vi "derivative_data view.vi"(8 "Y-column names":string[](array[string])=["col0"], 10 "column extension":string[](array[string])=["SCM1_2020Aug_AC.008.txt"], 11 "Graph array":cluster{"output":dbl[], "output":dbl[]}[](array[cluster])=[{"output"=array[450 elements], "output"=array[450 elements]}]) -> ()   [LabVIEW 2021]
uses:
  <vilib>/Analysis/1siggen.llb/Ramp Pattern by Samples.vi
  <vilib>/Analysis/NI_AALBase.lvlib
  <vilib>/gmath/NI_Gmath.lvlib
  <vilib>/Analysis/NI_AALPro.lvlib
panel:
  in  "iteration Number":i32=2
  in  "smooth factor":i32=121
  in  "method":u16(ring)=2 items=["2nd Order Central", "4th Order Central", "Forward", "Backward"]
  out "error code":i32
  out "bkg and subtracted data":cluster{"xi used":dbl[], "Integral X":dbl[]}[](graph)
  in  "remove bkg":bool=TRUE
  in  "Bbkg final":dbl=5.0 format="%.2f"
  in  "Bbkg initial":dbl=4.0 format="%.2f"
  in  "poly. order":i32=2
  in  "bkg removal method":enum16{"polynomial", "Cheby poly"}(ring)
  in  "export":T1(ring)=enum."write to clipboard"
  out "raw data":T2(graph)
  in  "interpol. method":i32(ring)=2 items=["nearest", "linear", "spline", "cubic Hermite", "Lagrange"]
  in  "stop":bool
  in  "use variables":bool
  in  "Interpolation #":i32=5000
  in  "export data":bool
  in  "smoothing factor":i32=3
  in  "final":dbl=5.0 format="%.2f"
  in  "init":dbl format="%.2f"
  out "dy/dx":cluster{"xi used":dbl[], "smoothed":dbl[]}[](graph)
  in  "variable":string="4.2\n3.5\n3"
  # "(0) Data are clipped defined by the 'init' and 'final'.\n(1) Boxcar averaging (use 'smoothing factor' for adjustment)\n(3) Background removal if necessary. Background removal is done by polynomial (normal or Chebychev).\n            i) fitting is done for the range given by 'Bbkg init' and 'Bbkg final'.\n            ii) the background curve is extended to the whole data range."
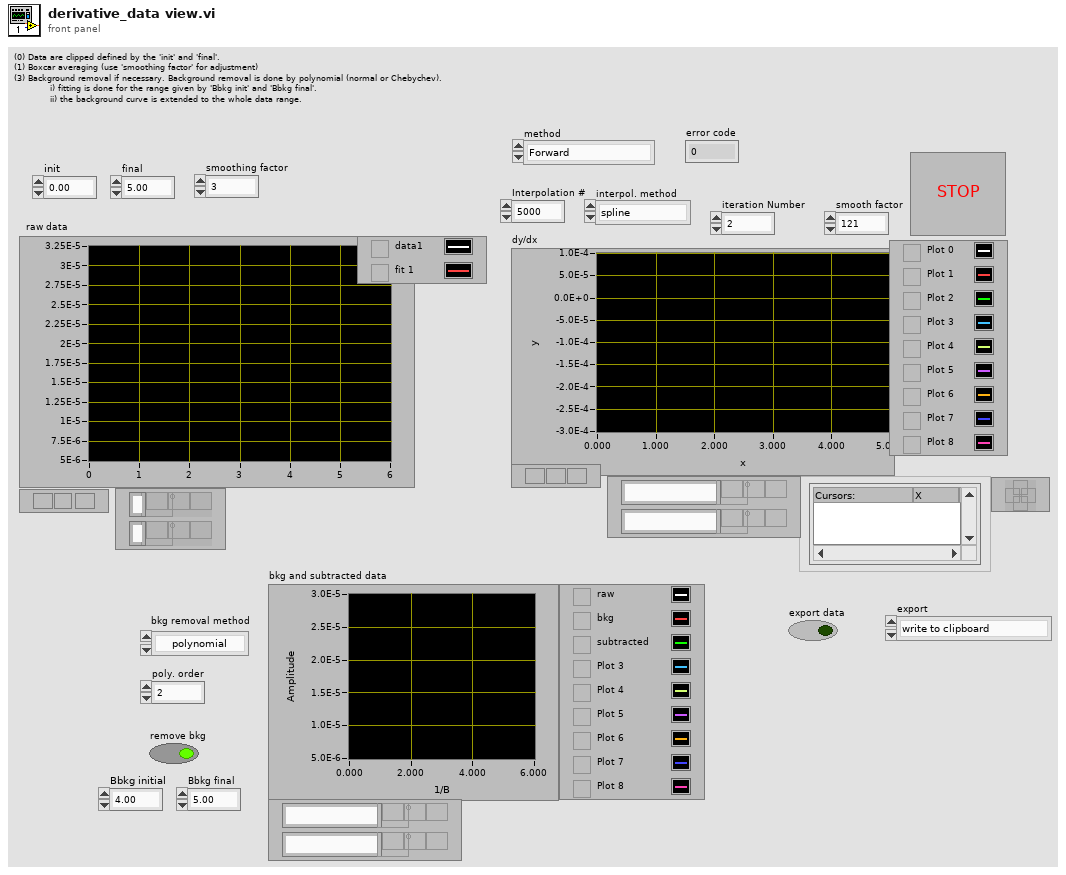
[diagram p1: front panel]
types:
  T1 = enum16{"Save as Ascill file", "write to clipboard", "write to Igor ITX file"}
  T2 = cluster{"Ramp Pattern":dbl[], "Power Spectrum":dbl[]}[]
  T3 = enum16{"Save as Ascill file", "write to clipboard", "do not export"}
  T4 = cluster{"all rows":dbl[], "extended data":dbl[]}[]
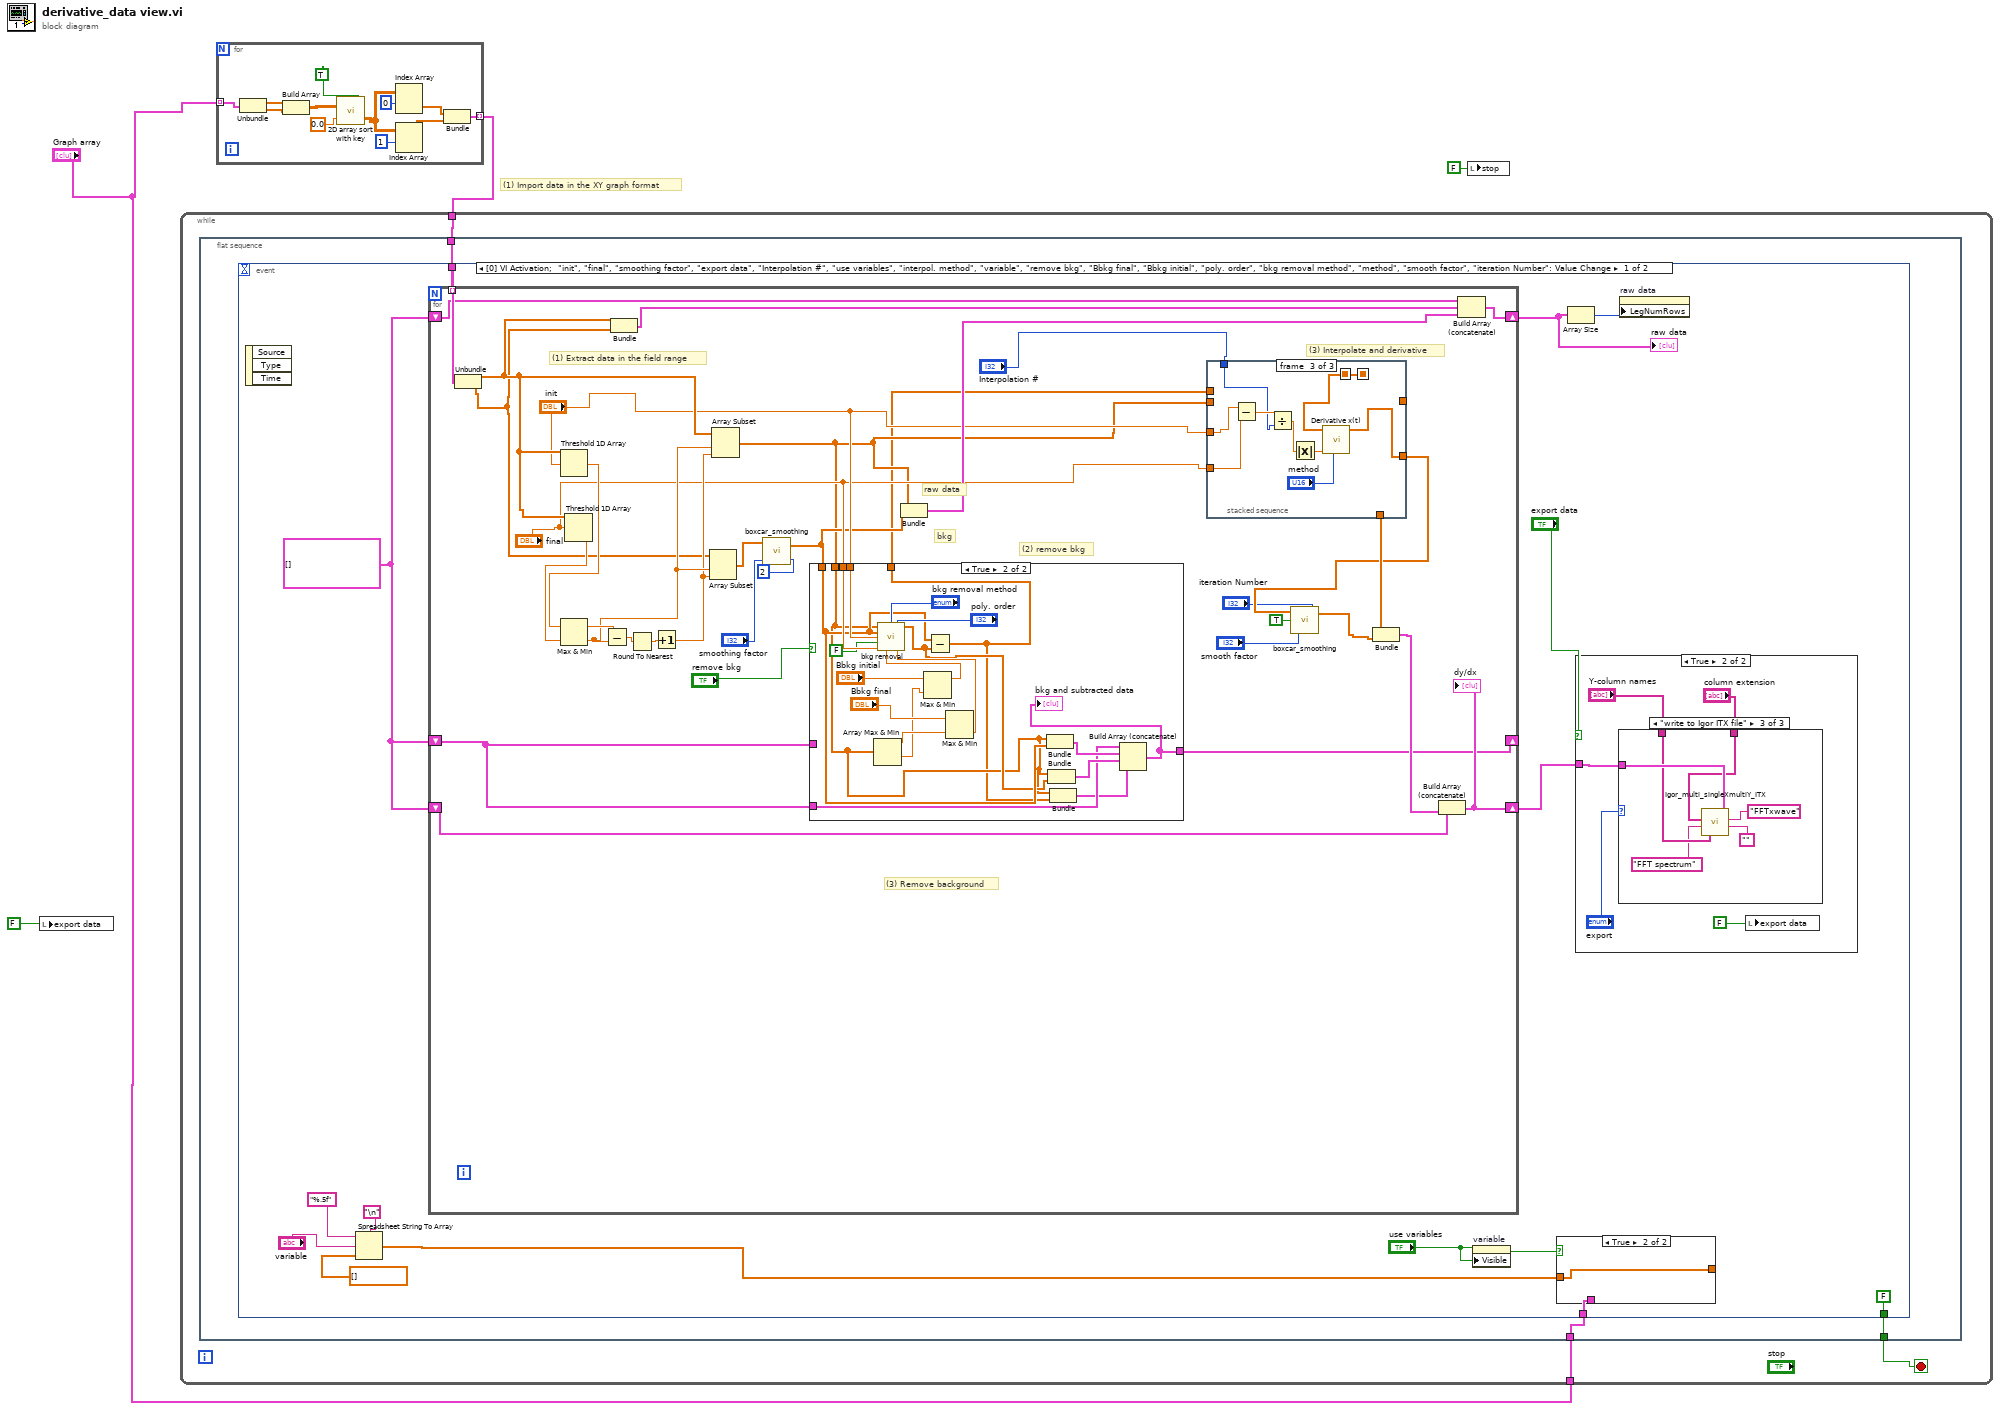
[diagram p0: block diagram]
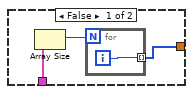
[diagram p2: hidden frame]
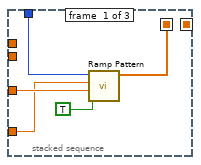
[diagram p4: hidden frame]
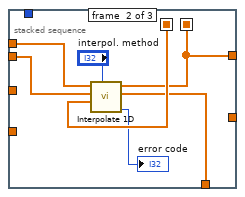
[diagram p5: hidden frame]
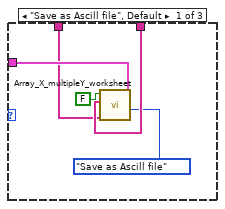
[diagram p7: hidden frame]
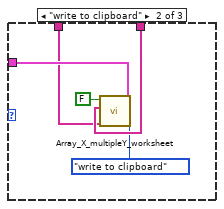
[diagram p8: hidden frame]
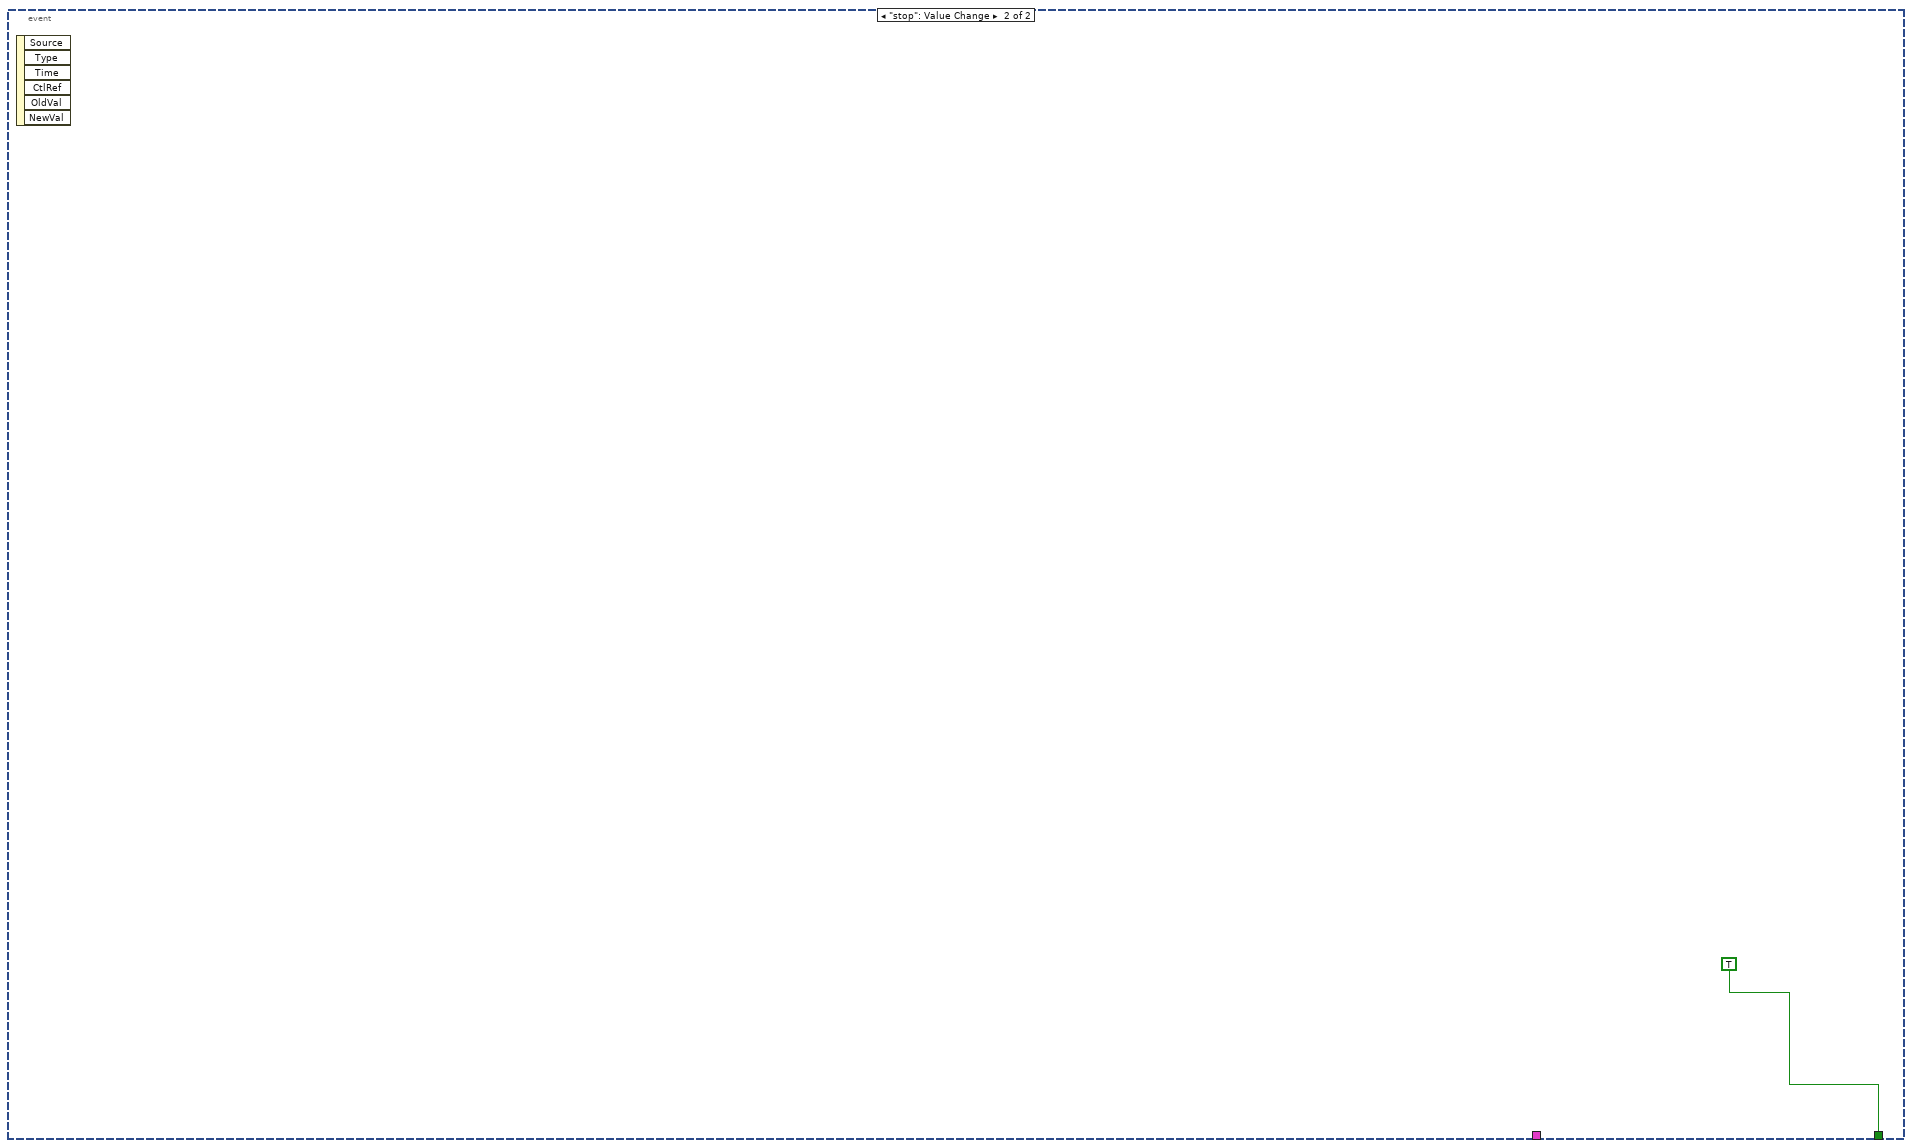
[diagram p9: hidden frame]
diagram:
  # "(1) Import data in the XY graph format"
  n1 = local write "export data"(FALSE ("export spectrum")) -> ()
  n2 = for {
    tunnel: "Graph array" -> [w16] mode=indexing
    tunnel: [w5] -> w3 mode=indexing
    n3 = Unbundle(w16) -> ("output"=w14:dbl[], "output"=w13:dbl[])
    n4 = Build Array(w14, w13) -> (w12:dbl[][])
    n5 = call "2D array sort with key.vi"("ascending"=TRUE, "key row"=0.0, "input"=w12) -> ("output"=w10:dbl[][])
    n6 = Index Array(array=w10, index (row)=0) -> (element=w7:dbl[])  [unwired: 1 in]
    n7 = Index Array(array=w10, index (row)=1) -> (element=w6:dbl[])  [unwired: 1 in]
    n8 = Bundle("output"=w7, "output"=w6) -> (w5:cluster{"output":dbl[], "output":dbl[]})  [unwired: 1 in]
  }
  n9 = while {
    tunnel: w3 -> [w19]
    tunnel: "Graph array" -> [w18]
    stop <- w17 stop-if-true
    n10 = flat-sequence {
      tunnel: w19 -> [w22]
      tunnel: w18 -> [w21]
      tunnel: [w20] -> w17
      frame #0 {
        n11 = event shown="[0] VI Activation;  \"init\", \"final\", \"smoothing factor\", \"export data\", \"Interpolation #\", \"use variables\", \"interpol. method\", \"variable\", \"remove bkg\", \"Bbkg final\", \"Bbkg initial\", \"poly. order\", \"bkg removal method\", \"method\", \"smooth factor\", \"iteration Number\": Value Change" {
          selector: _ -> [_ _]
          dyn-events: _ -> [_ _]
          timeout: _ -> [_ _]
          tunnel: w22 -> [w31 _]
          tunnel: w21 -> [w29 _]
          tunnel: [FALSE ("stop (press twice)") TRUE ("stop (press twice)")] -> w20
          event VI Activation; "init", "final", "smoothing factor", "export data", "Interpolation #", "use variables", "interpol. method", "variable", "remove bkg", "Bbkg final", "Bbkg initial", "poly. order", "bkg removal method", "method", "smooth factor", "iteration Number": Value Change {
            w23 = cluster{"all rows":sgl[], "all rows":sgl[]}[] []
            n12 = event-data() -> ()  [unwired: 1 in, 3 out]
            n13 = Spreadsheet String To Array(delimiter (Tab)="\n", format string="%.5f", spreadsheet string="variable", array type (2D Dbl)=dbl[] []) -> (array=w30:dbl[])
            n14 = for {
              shift-right: [w68] -> w24
              shift-left: w23 -> [w75]
              tunnel: w31 -> [w67] mode=indexing
              shift-right: [w65] -> w28
              shift-left: w23 -> [w64]
              shift-right: [w50] -> _
              shift-left: w23 -> [w49]
              # "(2) remove bkg"
              # "(3) Interpolate and derivative"
              # "(3) Remove background"
              # "(1) Extract data in the field range"
              # "bkg"
              # "raw data"
              n15 = Unbundle(w67) -> ("output"=w63:dbl[], "output"=w60:dbl[])
              n16 = Threshold 1D Array(2:"init", 3:w63) -> (0:w74:dbl)  [unwired: 1 in]
              n17 = Threshold 1D Array(2:"final", 3:w63) -> (0:w73:dbl)  [unwired: 1 in]
              n18 = Max & Min(x=w74, y=w73) -> (max(x,y)=w72:dbl, min(x,y)=w70:dbl)
              n19 = Subtract(x=w72, y=w70) -> (x-y=w71:dbl)
              n20 = Bundle("output"=w63, "output"=w60) -> (w62:cluster{"output":dbl[], "output":dbl[]})  [unwired: 1 in]
              n21 = Round To Nearest(number=w71) -> (nearest integer value=w76:dbl)
              n22 = Increment(x=w76) -> (x+1=w69:dbl)
              n23 = Array Subset(array=w60, index=w70, length=w69) -> (w59:dbl[])
              n24 = Array Subset(array=w63, index=w70, length=w69) -> (w48:dbl[])
              n25 = call "boxcar_smoothing.vi"("iteration Number"=2, "smooth factor"="smoothing factor", "raw data"=w59) -> ("smoothed"=w51:dbl[])  [unwired: 1 in]
              n26 = case shown="True" "remove bkg" {
                tunnel: w48 -> [_ w80]
                tunnel: w51 -> [w78 w87]
                tunnel: "init" -> [_ w98]
                tunnel: "final" -> [_ w97]
                tunnel: [w78 w79] -> w47
                tunnel: [w77 w82] -> w50
                tunnel: w49 -> [_ w83]
                tunnel: w49 -> [w77 _]
                frame False {
                }
                frame True {
                  n27 = Array Max & Min(array=w80) -> (max value=w92:dbl, min value=w91:dbl)  [unwired: 2 out]
                  n28 = Max & Min(x="Bbkg initial", y=w91) -> (max(x,y)=w88:dbl)  [unwired: 1 out]
                  n29 = Max & Min(x="Bbkg final", y=w92) -> (min(x,y)=w89:dbl)  [unwired: 1 out]
                  n30 = call "bkg removal.vi"("Bfield"=w80, "bkg removal method"="bkg removal method", "poly. order"="poly. order", "Data"=w87, "B initial"=w98, "inverse"=FALSE, "B final"=w97, "Bbkg initial"=w88, "Bbkg final"=w89) -> ("extended data"=w86:dbl[])  [unwired: 4 in, 2 out]
                  n31 = Subtract(x=w87, y=w86) -> (x-y=w79:dbl[])
                  n32 = Bundle(w80, "smoothed"=w87) -> (w85:cluster{dbl[], "smoothed":dbl[]})  [unwired: 1 in]
                  n33 = Bundle(w80, "extended data"=w86) -> (w84:cluster{dbl[], "extended data":dbl[]})  [unwired: 1 in]
                  n34 = Bundle(w80, w79) -> (w81:cluster{dbl[], dbl[]})  [unwired: 1 in]
                  n35 = Build Array (concatenate)(w83, w85, w84, w81) -> (w82:T4)
                  "bkg and subtracted data" <- w82
                }
              }
              n36 = Bundle(w48, "smoothed"=w51) -> (w61:cluster{dbl[], "smoothed":dbl[]})  [unwired: 1 in]
              n37 = stacked-sequence {
                seq-local: [w99 _ _] -> [_ w108 _]
                seq-local: [_ w105 _] -> [_ _ w115]
                tunnel: w47 -> [_ w110 _]
                tunnel: w48 -> [_ w107 _]
                tunnel: "Interpolation #" -> [w103 _ w116]
                tunnel: "init" -> [w102 _ w119]
                tunnel: "final" -> [w101 _ w118]
                tunnel: [_ _ w113] -> w46
                tunnel: [_ w106 _] -> w56
                tunnel: [_ w105 _] -> _
                frame #0 {
                  n38 = call-poly <vilib>:"Ramp Pattern.vi"("exclude end?"=TRUE, "start"=w102, "end"=w101, "samples"=w103) -> ("Ramp Pattern"=w99:dbl[])  [unwired: 6 in, 1 out]
                }
                frame #1 {
                  n39 = call <vilib>:"Interpolate 1D.vi"("method"="interpol. method", "xi"=w108, "X"=w107, "Y"=w110) -> ("error"=→"error code":i32, "xi used"=w106:dbl[], "yi"=w105:dbl[])  [unwired: 5 in]
                }
                frame #2 {
                  n40 = Subtract(x=w119, y=w118) -> (x-y=w117:dbl)
                  n41 = Divide(x=w117, y=w116) -> (x/y=w114:dbl)
                  n42 = Absolute Value(x=w114) -> (abs(x)=w112:dbl)
                  n43 = call <vilib>:"Derivative x(t).vi"("method"="method", "dt"=w112, "X"=w115) -> ("dX/dt"=w113:dbl[])  [unwired: 7 in, 1 out]
                }
              }
              n44 = call "boxcar_smoothing.vi"("iteration Number"="iteration Number", "smooth factor"="smooth factor", "remonve NaN"=TRUE, "raw data"=w46) -> ("smoothed"=w42:dbl[])
              n45 = Bundle("xi used"=w56, "smoothed"=w42) -> (w55:cluster{"xi used":dbl[], "smoothed":dbl[]})  [unwired: 1 in]
              n46 = Build Array (concatenate)(w75, w55) -> (w68:cluster{"xi used":dbl[], "smoothed":dbl[]}[])
              "dy/dx" <- w68
              n47 = Build Array (concatenate)(w64, w62, w61) -> (w65:cluster{"output":dbl[], "smoothed":dbl[]}[])
            }
            "raw data" <- w28
            n48 = property on="variable" class="Str"("Visible"="use variables") -> ()  [unwired: 2 in, 2 out]
            n49 = case shown="True" "use variables" {
              tunnel: w30 -> [_ w41]
              tunnel: [w38 w41] -> _
              tunnel: w29 -> [w37 _]
              frame False {
                n50 = Array Size(array=w37) -> (size(s)=w39:i32)
                n51 = for {
                  N: w39 -> [_]
                  tunnel: [w40] -> w38 mode=indexing
                  i -> [w40]
                }
              }
              frame True {
              }
            }
            n52 = Array Size(array=w28) -> (size(s)=w27:i32)
            n53 = case shown="True" "export data" {
              tunnel: w24 -> [_ w123]
              frame False {
              }
              frame True {
                n54 = case shown="\"write to Igor ITX file\"" "export" {
                  tunnel: w123 -> [w129 w134 w140]
                  tunnel: "column extension" -> [w127 w132 w139]
                  tunnel: "Y-column names" -> [w126 w131 w138]
                  frame "Save as Ascill file", Default {
                    n55 = call "Array_X_multipleY_worksheet.vi"("export"=T3."Save as Ascill file", "graph file"=w129, "Y-column names"=w126, "column extension"=w127, "Sort?"=FALSE) -> ()  [unwired: 3 in, 2 out]
                  }
                  frame "write to clipboard" {
                    n56 = call "Array_X_multipleY_worksheet.vi"("export"=T3."write to clipboard", "graph file"=w134, "Y-column names"=w131, "column extension"=w132, "Sort?"=FALSE) -> ()  [unwired: 3 in, 2 out]
                  }
                  frame "write to Igor ITX file" {
                    n57 = call "Igor_multi_singleXmultiY_ITX.vi"("message"="", "x-column name"="FFTxwave", "graph file"=w140, "Y-column names"=w138, "window name"="FFT spectrum", "column extension"=w139) -> ()  [unwired: 1 in, 1 out]
                  }
                }
                n58 = local write "export data"(FALSE ("export spectrum")) -> ()
              }
            }
            n59 = property on="raw data" class="XYGraph (strict)"("LegNumRows"=w27) -> ()  [unwired: 2 in, 2 out]
          }
          event "stop": Value Change {
            n60 = event-data() -> ()  [unwired: 1 in, 6 out]
          }
        }
      }
    }
  }
  n61 = local write "stop"(FALSE ("stop")) -> ()
